vi "ABB Test Bearing Inspection.vi"() -> ()   [LabVIEW 2017]
uses:
  ABB global.vi
panel:
  in  "A/R1 8":bool caption="Accept"
  out "Criteria 8":string
  in  "A/R1 7":bool caption="Accept"
  out "Criteria 7":string
  in  "A/R1 6":bool caption="Accept"
  out "Criteria 6":string
  in  "A/R1 5":bool caption="Accept"
  out "Criteria 5":string
  in  "A/R1 4":bool caption="Accept"
  out "Criteria 4":string
  in  "A/R1 3":bool caption="Accept"
  out "Criteria 3":string
  in  "A/R1 2":bool caption="Accept"
  out "Criteria 2":string
  in  "A/R1":bool caption="Accept"
  out "Criteria 1":string
  out "Picture 8":picture
  out "Picture 7":picture
  out "Picture 6":picture
  out "Picture 5":picture
  out "Picture 4":picture
  out "Picture 3":picture
  out "Picture 2":picture
  out "Picture 1":picture
  out "Serial number":string
  out "W.O number":string
  out "Timedate":string
  in  "Exit":bool
  # "Bearing Inspection"
  # "?"
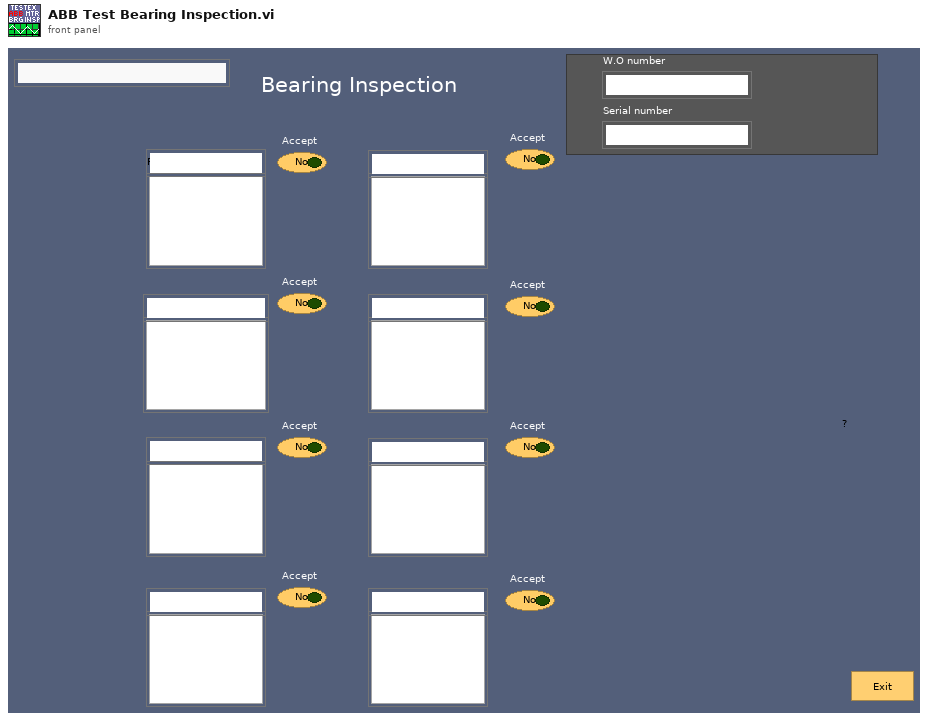
[diagram p1: front panel]
types:
  T1 = cluster{"Simulate Norma":bool, "Norma 5000 Address":u8, "WebDaq IP Address":string, "Simulate cDAQ":bool}
  T2 = typedef "imagedata.ctl" = cluster{"image type":i32, "image depth":i32, "image":u8[], "mask":u8[], "colors":u32[], "Rectangle":cluster{"left":i16, "top":i16, "right":i16, "bottom":i16}}
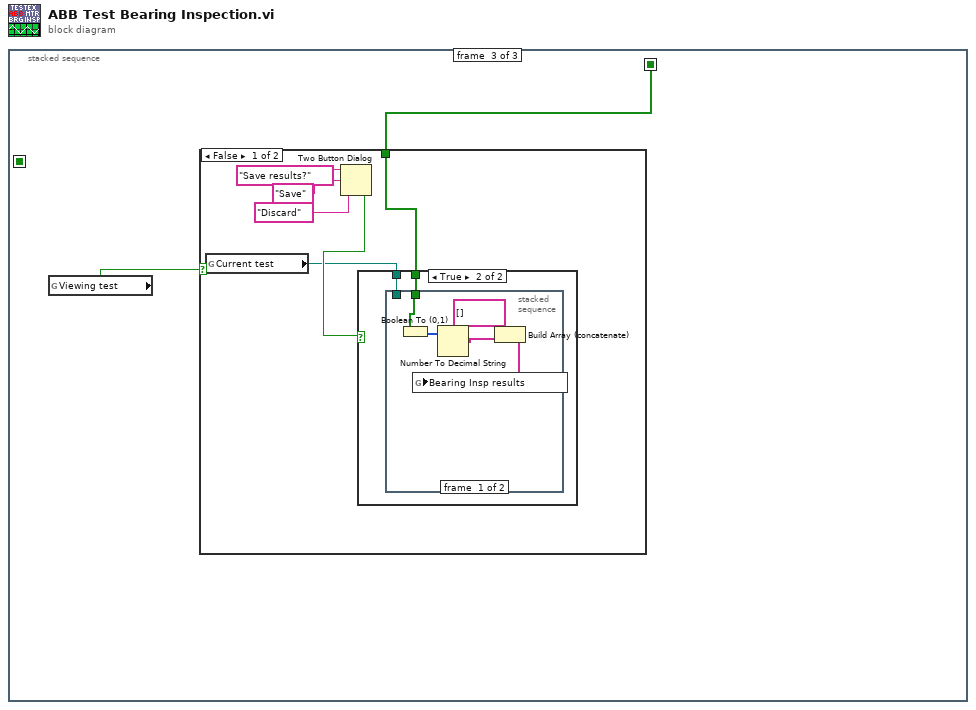
[diagram p0: block diagram]
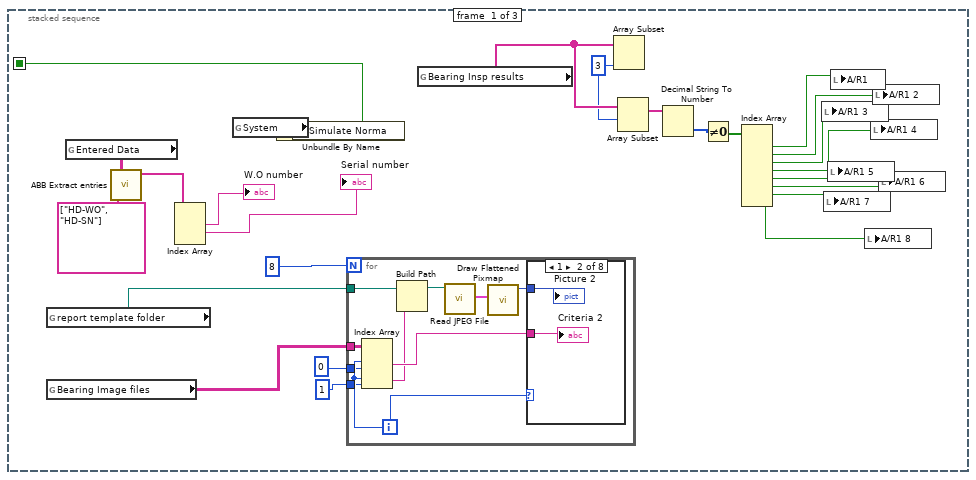
[diagram p2: hidden frame]
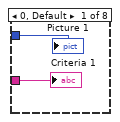
[diagram p3: hidden frame]
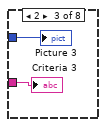
[diagram p4: hidden frame]
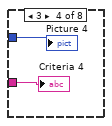
[diagram p5: hidden frame]
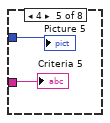
[diagram p6: hidden frame]
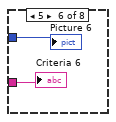
[diagram p7: hidden frame]
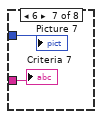
[diagram p8: hidden frame]
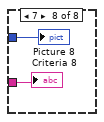
[diagram p9: hidden frame]
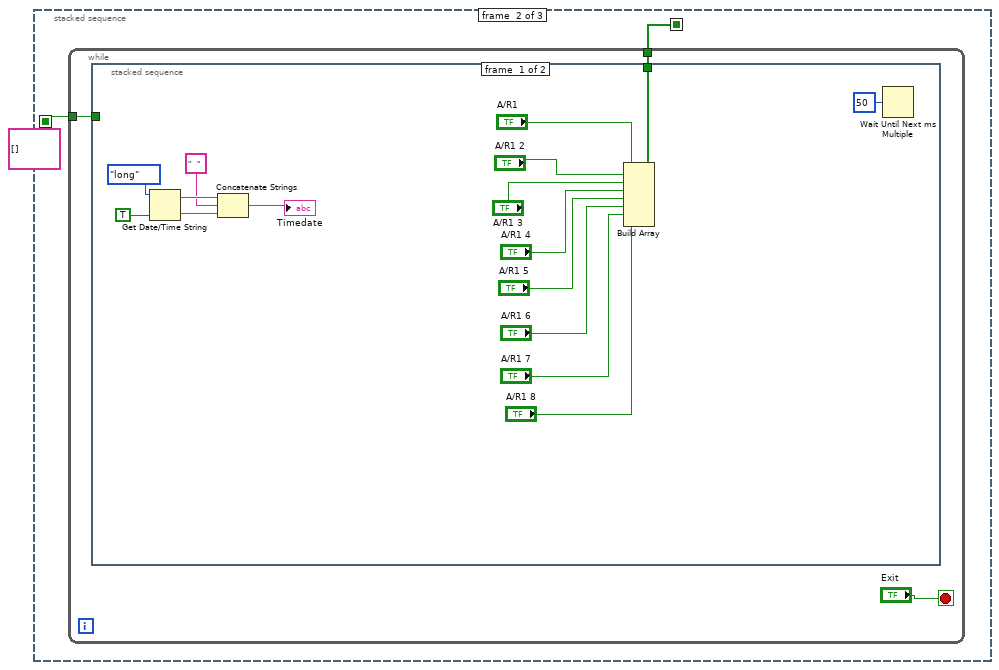
[diagram p10: hidden frame]
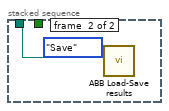
[diagram p13: hidden frame]
diagram:
  n1 = stacked-sequence {
    seq-local: [w24 _ _] -> [_ w53 _]
    seq-local: [_ w52 _] -> [_ _ w74]
    frame #0 {
      w16 = 3 ("length")
      n2 = global read "ABB global.vi" "report template folder"() -> (w18:path)
      n3 = global read "ABB global.vi" "Bearing Image files"() -> (w3:string[][])
      n4 = global read "ABB global.vi" "Entered Data"() -> (w21:string[][])
      n5 = call "ABB Extract entries.vi"("Entry IDs"=string[] ["HD-WO", "HD-SN"], "Entry table in"=w21) -> ("Selected Entries"=w20:string[])  [unwired: 9 in]
      n6 = Index Array(array=w20) -> (element #1=→"W.O number":string, element #2=→"Serial number":string)  [unwired: 3 in, 1 out]
      n7 = global read "ABB global.vi" "System"() -> (w25:T1)
      n8 = Unbundle By Name(w25) -> ("Simulate Norma"=w24:bool)
      n9 = for {
        N: 8 -> [_]
        tunnel: w18 -> [w35]
        tunnel: w3 -> [w31]
        tunnel: 0 ("disabled index (col)") -> [w27]
        tunnel: 1 ("index (col)") -> [w26]
        i -> [w28]
        n10 = Index Array(array=w31, index (row) #1=w28, index (col) #1=w27, index (row) #2=w28, index (col) #2=w26) -> (element #1=w30:string, element #2=w29:string)
        n11 = Build Path(base path=w35, name or relative path=w29) -> (appended path=w33:path)
        n12 = call <vilib>:"Read JPEG File.vi"("path to JPEG file"=w33) -> ("image data"=w34:T2)  [unwired: 8 in, 2 out]
        n13 = call <vilib>:"Draw Flattened Pixmap.vi"("image data"=w34) -> ("new picture"=w32:picture)  [unwired: 8 in]
        n14 = case shown="1" w28 {
          tunnel: w30 -> [w37 w39 w41 w43 w45 w47 w49 w51]
          tunnel: w32 -> [w36 w38 w40 w42 w44 w46 w48 w50]
          frame 0, Default {
            "Criteria 1" <- w37
            "Picture 1" <- w36
          }
          frame 1 {
            "Criteria 2" <- w39
            "Picture 2" <- w38
          }
          frame 2 {
            "Criteria 3" <- w41
            "Picture 3" <- w40
          }
          frame 3 {
            "Criteria 4" <- w43
            "Picture 4" <- w42
          }
          frame 4 {
            "Criteria 5" <- w45
            "Picture 5" <- w44
          }
          frame 5 {
            "Criteria 6" <- w47
            "Picture 6" <- w46
          }
          frame 6 {
            "Criteria 7" <- w49
            "Picture 7" <- w48
          }
          frame 7 {
            "Criteria 8" <- w51
            "Picture 8" <- w50
          }
        }
      }
      n15 = global read "ABB global.vi" "Bearing Insp results"() -> (w17:string[])
      n16 = Array Subset(array=w17, length=w16) -> ()  [unwired: 1 in, 1 out]
      n17 = Array Subset(array=w17, index=w16) -> (w15:string[])  [unwired: 1 in]
      n18 = Decimal String To Number(string=w15) -> (number=w14:i32[])  [unwired: 2 in, 1 out]
      n19 = Not Equal To 0?(x=w14) -> (x != 0?=w13:bool[])
      n20 = Index Array(array=w13) -> (element #1=w12:bool, element #2=w11:bool, element #3=w10:bool, element #4=w9:bool, element #5=w8:bool, element #6=w7:bool, element #7=w6:bool, element #8=w5:bool)  [unwired: 8 in]
      n21 = local write "A/R1 3"(w10) -> ()
      n22 = local write "A/R1 7"(w6) -> ()
      n23 = local write "A/R1 5"(w8) -> ()
      n24 = local write "A/R1"(w12) -> ()
      n25 = local write "A/R1 8"(w5) -> ()
      n26 = local write "A/R1 4"(w9) -> ()
      n27 = local write "A/R1 2"(w11) -> ()
      n28 = local write "A/R1 6"(w7) -> ()
    }
    frame #1 {
      (unwired) string[][] [] ("Cooling Curve Data")
      n29 = while {
        tunnel: w53 -> [w55]
        tunnel: [w54] -> w52
        stop <- "Exit" stop-if-true
        n30 = stacked-sequence {
          tunnel: w55 -> [_ _]
          tunnel: [w57 _] -> w54
          frame #0 {
            n31 = Get Date/Time String(date format (0)=enum16{"short", "long", "abbreviated"}."long", want seconds? (F)=TRUE) -> (date string=w70:string, time string=w69:string)  [unwired: 1 in]
            n32 = Concatenate Strings(w70, "   ", w69) -> (→"Timedate":string)
            n33 = Build Array("A/R1", "A/R1 2", "A/R1 3", "A/R1 4", "A/R1 5", "A/R1 6", "A/R1 7", "A/R1 8") -> (w57:bool[])
            n34 = Wait Until Next ms Multiple(millisecond multiple=u32 50) -> ()  [unwired: 1 out]
          }
          frame #1 {
          }
        }
      }
    }
    frame #2 {
      n35 = global read "ABB global.vi" "Viewing test"() -> (w73:bool)
      n36 = case shown="False" w73 {
        tunnel: w74 -> [w77 _]
        frame False {
          n37 = global read "ABB global.vi" "Current test"() -> (w78:path)
          n38 = Two Button Dialog(message="Save results?", 1:"Discard" ("F button name (\"Cancel\")"), 2:"Save" ("T button name (\"OK\")")) -> (T button?=w79:bool)
          n39 = case shown="True" w79 {
            tunnel: w78 -> [_ w82]
            tunnel: w77 -> [_ w81]
            frame False {
            }
            frame True {
              n40 = stacked-sequence {
                tunnel: w82 -> [_ w88]
                tunnel: w81 -> [w87 _]
                frame #0 {
                  n41 = Boolean To (0,1)(Boolean=w87) -> (0, 1=w86:i16[])
                  n42 = Number To Decimal String(number=w86) -> (decimal integer string=w85:string[])  [unwired: 1 in]
                  n43 = Build Array (concatenate)(string[] [] ("array"), w85) -> (w84:string[])
                  n44 = global write "ABB global.vi" "Bearing Insp results"(w84) -> ()
                }
                frame #1 {
                  n45 = call "ABB Load-Save results.vi"("Path"=w88, "Mode"=enum16{"LOAD", "Save"}."Save") -> ()  [unwired: 10 in]
                }
              }
            }
          }
        }
        frame True {
        }
      }
    }
  }
